vi "PID.vi"() -> ()   [LabVIEW 2018]
panel:
  in  "derivative time (Td, min)":dbl
  in  "integral time (Ti, min)":dbl
  in  "proportional gain (Kc)":dbl
  in  "output range":cluster{"output high":dbl, "output low":dbl}={"output high"=100.0, "output low"=-100.0} {"output low" format="%.2f"; "output high" format="%.2f"}
  out "output":dbl format="%.2f"
  in  "dt (s)":dbl=-1.0 format="%.3f"
  in  "setpoint":dbl format="%.2f"
  in  "process variable":dbl format="%.2f"
  out "dt out (s)":dbl format="%.3f"
  in  "reinitialize? (F)":bool
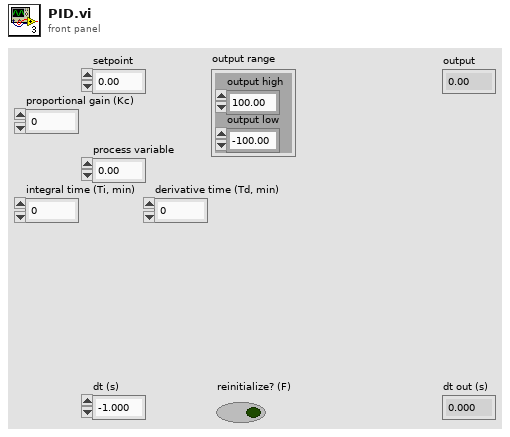
[diagram p1: front panel]
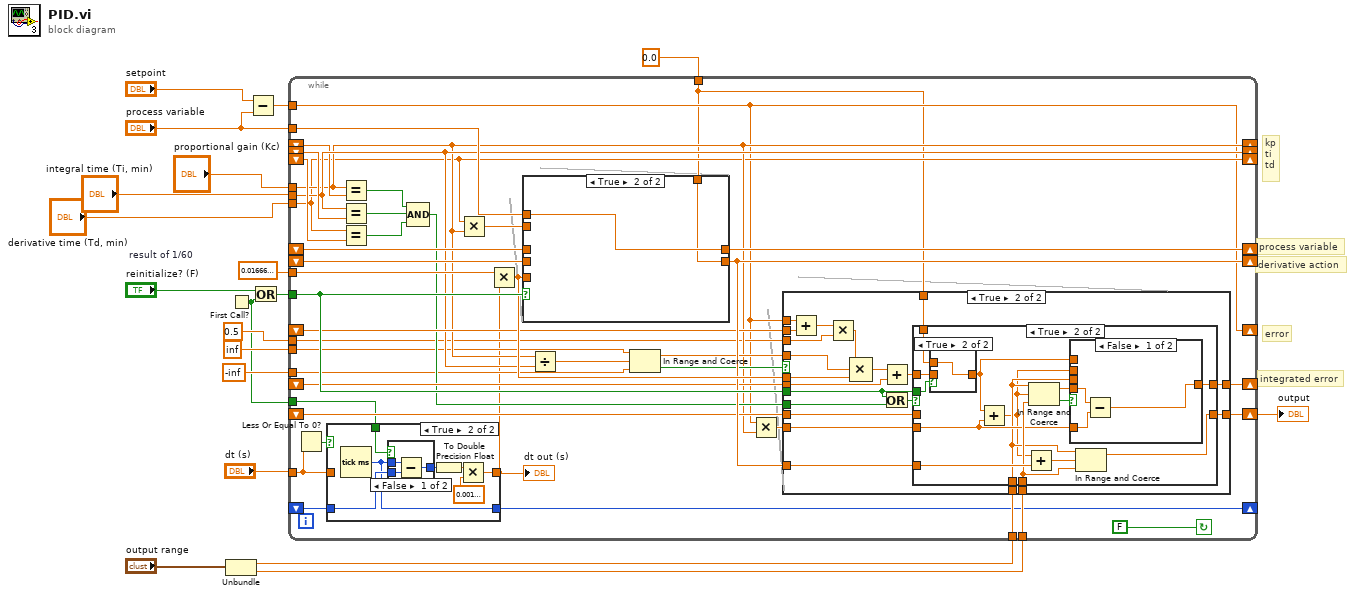
[diagram p0: block diagram]
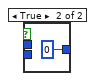
[diagram p3: hidden frame]
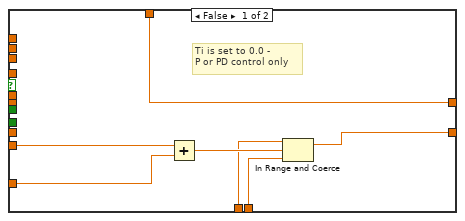
[diagram p4: hidden frame]
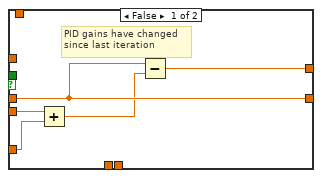
[diagram p5: hidden frame]
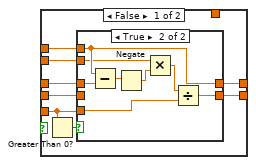
[diagram p8: hidden frame]
diagram:
  w16 = 0.016666666666666666  # result of 1/60
  # "derivative action"
  # "process variable"
  # "kp\nti\ntd"
  # "error"
  # "integrated error"
  n1 = Unbundle("output range") -> ("output high"=w18:dbl, "output low"=w17:dbl)
  n2 = First Call?() -> (First Call?: T/F=w4:bool)
  n3 = Subtract(x="setpoint", y="process variable") -> (x-y=w6:dbl)
  n4 = Or(x="reinitialize? (F)", y=w4) -> (x .or. y?=w19:bool)
  n5 = while {
    tunnel: w19 -> [w61]
    shift-left: _ -> [w23]
    shift-right: [w24] -> _
    shift-right: [w33] -> _
    shift-left: _ -> [w34]
    shift-right: [w35] -> _
    shift-left: _ -> [w58]
    shift-right: [w28] -> _
    shift-left: _ -> [w59]
    tunnel: "proportional gain (Kc)" -> [w33]
    tunnel: "integral time (Ti, min)" -> [w35]
    tunnel: "derivative time (Td, min)" -> [w28]
    tunnel: "dt (s)" -> [w22]
    tunnel: w18 -> [w54]
    tunnel: w17 -> [w53]
    tunnel: "process variable" -> [w52]
    shift-right: [w51] -> _
    shift-left: _ -> [w50]
    shift-right: [w49] -> _
    shift-left: _ -> [w41]
    shift-right: [w48] -> w10
    shift-left: _ -> [w47]
    shift-right: [w27] -> _
    shift-left: _ -> [w46]
    shift-right: [w45] -> _
    shift-left: _ -> [w44]
    tunnel: w16 -> [w38]
    tunnel: 0.5 ("y") -> [w32]
    tunnel: inf ("upper limit") -> [w30]
    tunnel: -inf ("lower limit") -> [w31]
    tunnel: w6 -> [w27]
    tunnel: 0.0 -> [w26]
    tunnel: w4 -> [w20]
    stop <- FALSE continue-if-true
    n6 = Less Or Equal To 0?(x=w22) -> (x <= 0?=w21:bool)
    n7 = case shown="True" w21 {
      tunnel: [w63 w67] -> w25
      tunnel: w23 -> [w62 w66]
      tunnel: [w62 w65] -> w24
      tunnel: w22 -> [w63 _]
      tunnel: w20 -> [_ w64]
      frame False {
      }
      frame True {
        n8 = Tick Count (ms)() -> (millisecond timer value=w65:u32)
        n9 = case shown="False" w64 {
          tunnel: [w73 u32 0] -> w69
          tunnel: w66 -> [w72 _]
          tunnel: w65 -> [w71 _]
          frame False {
            n10 = Subtract(x=w71, y=w72) -> (x-y=w73:u32)
          }
          frame True {
          }
        }
        n11 = To Double Precision Float(number=w69) -> (double precision float=w68:dbl)
        n12 = Multiply(x=w68, y=0.0010000000474974513) -> (x*y=w67:dbl)
      }
    }
    "dt out (s)" <- w25
    n13 = Equal?(x=w33, y=w34) -> (x = y?=w56:bool)
    n14 = Equal?(x=w35, y=w58) -> (x = y?=w55:bool)
    n15 = Equal?(x=w28, y=w59) -> (x = y?=w57:bool)
    n16 = Compound Arithmetic op=AND(w56, w55, w57) -> (w36:bool)
    n17 = Multiply(x=w28, y=w33) -> (x*y=w40:dbl)
    n18 = Multiply(x=w38, y=w25) -> (x*y=w60:dbl)
    n19 = case shown="True" w61 {
      tunnel: w50 -> [w135 _]
      tunnel: w40 -> [w132 _]
      tunnel: w52 -> [w134 w147]
      tunnel: [w131 w147] -> w51
      tunnel: [w133 w146] -> w49
      tunnel: w41 -> [w129 _]
      tunnel: w60 -> [w128 _]
      tunnel: w26 -> [_ w146]
      frame False {
        n20 = Greater Than 0?(x=w128) -> (x > 0?=w130:bool)
        n21 = case shown="True" w130 {
          tunnel: w135 -> [w137 w143]
          tunnel: w128 -> [_ w142]
          tunnel: w134 -> [_ w140]
          tunnel: [w136 w141] -> w133
          tunnel: w132 -> [_ w138]
          tunnel: [w137 w140] -> w131
          tunnel: w129 -> [w136 _]
          frame False {
            # "dt = 0 min"
          }
          frame True {
            n22 = Subtract(x=w140, y=w143) -> (x-y=w145:dbl)
            n23 = Negate(x=w145) -> (-x=w139:dbl)
            n24 = Multiply(x=w138, y=w139) -> (x*y=w144:dbl)
            n25 = Divide(x=w144, y=w142) -> (x/y=w141:dbl)
          }
        }
      }
      frame True {
      }
    }
    n26 = Divide(x=w33, y=w35) -> (x/y=w39:dbl)
    n27 = In Range and Coerce(upper limit=w30, x=w39, lower limit=w31) -> (coerced(x)=w43:dbl, In Range?=w42:bool)
    n28 = Multiply(x=w27, y=w33) -> (x*y=w37:dbl)
    n29 = case shown="True" w42 {
      tunnel: w27 -> [_ w101]
      tunnel: w46 -> [_ w102]
      tunnel: w44 -> [_ w97]
      tunnel: [w75 w92] -> w45
      tunnel: w43 -> [_ w90]
      tunnel: w37 -> [w80 w95]
      tunnel: [w81 w91] -> w48
      tunnel: w47 -> [_ w93]
      tunnel: w49 -> [w79 w89]
      tunnel: w61 -> [_ w88]
      tunnel: w36 -> [_ w87]
      tunnel: w60 -> [_ w86]
      tunnel: w54 -> [w77 w84]
      tunnel: w53 -> [w76 w85]
      tunnel: w32 -> [_ w83]
      tunnel: w26 -> [w75 w82]
      frame False {
        # "Ti is set to 0.0 -\nP or PD control only"
        n30 = Add(x=w80, y=w79) -> (x+y=w78:dbl)
        n31 = In Range and Coerce(upper limit=w77, x=w78, lower limit=w76) -> (coerced(x)=w81:dbl)  [unwired: 1 out]
      }
      frame True {
        n32 = Add(x=w101, y=w102) -> (x+y=w100:dbl)
        n33 = Multiply(x=w100, y=w83) -> (x*y=w99:dbl)
        n34 = Compound Arithmetic op=MULTIPLY(w99, w90, w86) -> (w98:dbl)
        n35 = Add(x=w98, y=w97) -> (x+y=w96:dbl)
        n36 = Or(x=w88, y=w87) -> (x .or. y?=w94:bool)
        n37 = case shown="True" w94 {
          tunnel: w96 -> [_ w115]
          tunnel: w95 -> [w105 w110]
          tunnel: w93 -> [w107 _]
          tunnel: w88 -> [_ w117]
          tunnel: [w106 w112] -> w92
          tunnel: [w107 w120] -> w91
          tunnel: w89 -> [w104 w119]
          tunnel: w85 -> [_ w118]
          tunnel: w84 -> [_ w109]
          tunnel: w82 -> [_ w116]
          frame False {
            # "PID gains have changed\nsince last iteration"
            n38 = Add(x=w105, y=w104) -> (x+y=w103:dbl)
            n39 = Subtract(x=w107, y=w103) -> (x-y=w106:dbl)
          }
          frame True {
            n40 = case shown="True" w117 {
              tunnel: w116 -> [_ w127]
              tunnel: [w126 w127] -> w114
              tunnel: w115 -> [w126 _]
              frame False {
              }
              frame True {
              }
            }
            n41 = Add(x=w114, y=w110) -> (x+y=w108:dbl)
            n42 = Add(x=w108, y=w119) -> (x+y=w121:dbl)
            n43 = In Range and Coerce(upper limit=w109, x=w108, lower limit=w118) -> (coerced(x)=w111:dbl, In Range?=w113:bool)
            n44 = case shown="False" w113 {
              tunnel: w114 -> [_ w125]
              tunnel: [w122 w125] -> w112
              tunnel: w111 -> [w124 _]
              tunnel: w110 -> [w123 _]
              tunnel: w109 -> [_ _]
              tunnel: w108 -> [_ _]
              frame False {
                n45 = Subtract(x=w124, y=w123) -> (x-y=w122:dbl)
              }
              frame True {
              }
            }
            n46 = In Range and Coerce(upper limit=w109, x=w121, lower limit=w118) -> (coerced(x)=w120:dbl)  [unwired: 1 out]
          }
        }
      }
    }
  }
  "output" <- w10
